vi "Generate-a.vi"(0 "Stop":bool, 11 "Error in":errorcluster) -> (4 "Numeric":dbl, 15 "Error out":errorcluster)   [LabVIEW 2020]
doc: "This VI is used to generate random number and send it to another VI with the help of global variable"
uses:
  SubVI/Stop Global Variable.vi
  SubVI/Numeric Global variable.vi
panel:
  # "This VI will generate random numbers and populate it to \nanother VI."
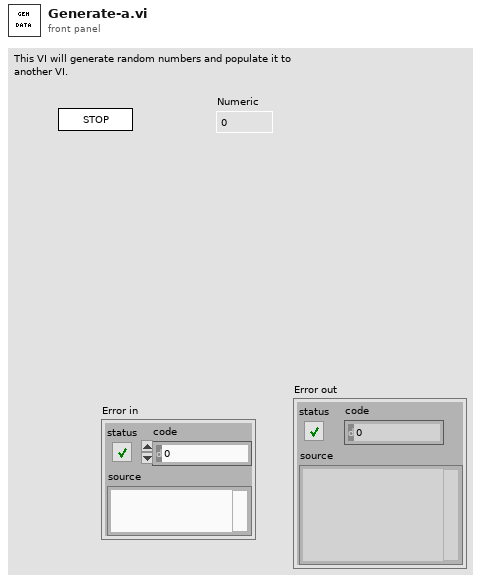
[diagram p1: front panel]
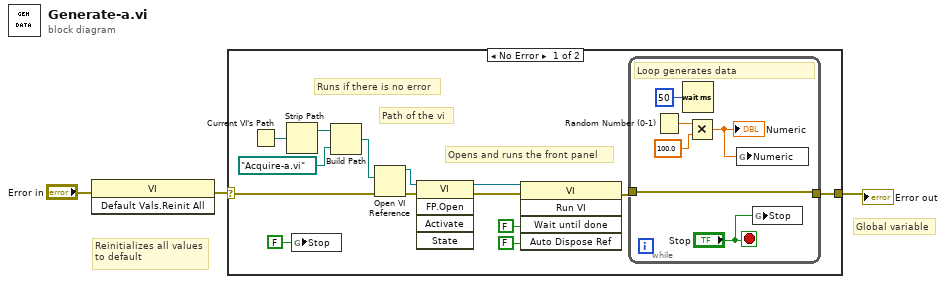
[diagram p0: block diagram]
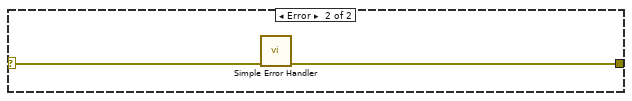
[diagram p2: hidden frame]
diagram:
  # "Global variable"
  # "Reinitializes all values\nto default"
  n1 = invoke class="VI" method="Default Vals.Reinit All"(error in="Error in") -> (error out=w2:errorcluster)  [unwired: 2 in, 2 out]
  n2 = case shown="No Error" w2 {
    selector: w2 -> [w14 w25]
    tunnel: [w13 w24] -> w3
    frame No Error {
      # "Opens and runs the front panel"
      # "Path of the vi"
      # "Runs if there is no error"
      n3 = Current VI's Path() -> (path=w17:path)
      n4 = Strip Path(path=w17) -> (stripped path=w16:path)  [unwired: 1 out]
      n5 = global write "Stop Global Variable.vi" "Stop"(FALSE ("Stop")) -> ()
      n6 = Build Path(base path=w16, name or relative path=path "Acquire-a.vi") -> (appended path=w12:path)
      n7 = Open VI Reference(vi path=w12, error in (no error)=w14) -> (vi reference=w10:refnum<vi>, error out=w11:errorcluster)  [unwired: 4 in]
      n8 = invoke class="VI" method="FP.Open"(reference=w10, error in=w11) -> (reference out=w9:refnum<vi>, error out=w8:errorcluster)  [unwired: 3 in, 3 out]
      n9 = invoke class="VI" method="Run VI"(reference=w9, error in=w8, "Wait until done"=FALSE ("Wait Until Done"), "Auto Dispose Ref"=FALSE ("Auto Dispose Reference")) -> (error out=w5:errorcluster)  [unwired: 1 in, 4 out]
      n10 = while {
        tunnel: [w19] -> w13
        tunnel: w5 -> [w19]
        stop <- "Stop" stop-if-true
        # "Loop generates data"
        n11 = Random Number (0-1)() -> (number: 0 to 1=w23:dbl)
        n12 = Wait (ms)(milliseconds to wait=u32 50) -> ()  [unwired: 1 out]
        n13 = Multiply(x=w23, y=100.0) -> (x*y=w20:dbl)
        "Numeric" <- w20
        n14 = global write "Numeric Global variable.vi" "Numeric"(w20) -> ()
        n15 = global write "Stop Global Variable.vi" "Stop"("Stop") -> ()
      }
    }
    frame Error {
      n16 = call <vilib>:"Simple Error Handler.vi"("error in (no error)"=w25) -> ("error out"=w24:errorcluster)  [unwired: 4 in, 4 out]
    }
  }
  "Error out" <- w3
